vi "WSVCAP SHL Host TL RFFE Write Cycle - Single DUT.vi"(0 "Data Out (Cycle Commands)":string[](array[string]), 5 "Post Command Delay":dbl[](array[numeric]) format="%#.0p s", 11 "error in":errorcluster, 12 "Log (T)":bool=TRUE, 13 "DUT":T2, 14 "FPGA":T1) -> (15 "error out":errorcluster)   [LabVIEW 2017]
uses:
  Type Defs/WSVCAP SHL DUT Number Enum.ctl
  Type Defs/WSVCAP SHL FPGA Enum.ctl
panel:
  out "Socket Mask":u64=1 format="%016x"
  out "RFFE Data Out":u8[][](array[numeric]) format="%02x"
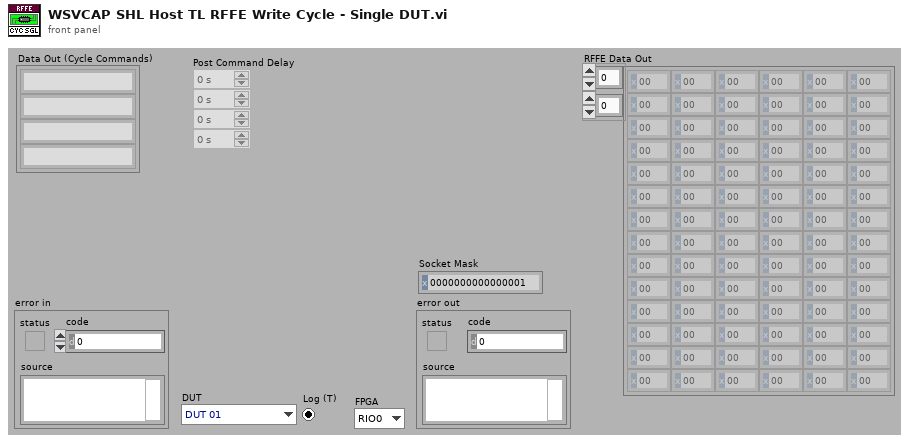
[diagram p1: front panel]
types:
  T1 = typedef "WSVCAP SHL FPGA Enum.ctl" = enum16{"RIO0", "RIO1"}
  T2 = typedef "WSVCAP SHL DUT Number Enum.ctl" = enum16{"DUT 01", "DUT 02", "DUT 03", "DUT 04", "DUT 05", "DUT 06", "DUT 07", "DUT 08", "DUT 09", "DUT 10", "DUT 11", "DUT 12", "DUT 13", "DUT 14", "DUT 15", "DUT 16", "DUT 17", "DUT 18", "DUT 19", "DUT 20", "DUT 21", "DUT 22", "DUT 23", "DUT 24", "DUT 25", "DUT 26", "DUT 27", "DUT 28", "DUT 29", "DUT 30", "DUT 31", "DUT 32", "DUT 33", "DUT 34", "DUT 35", "DUT 36", "DUT 37", "DUT 38", "DUT 39", "DUT 40", "DUT 41", "DUT 42", "DUT 43", "DUT 44", "DUT 45", "DUT 46", "DUT 47", "DUT 48", "DUT 49", "DUT 50", "DUT 51", "DUT 52", "DUT 53", "DUT 54", "DUT 55", "DUT 56", "DUT 57", "DUT 58", "DUT 59", "DUT 60", "DUT 61", "DUT 62", "DUT 63", "DUT 64"}
  T3 = typedef "WSVCAP SHL Core System Cluster.ctl" = cluster{"Settings":T4, "FPGA Resource":tag, "Online":bool, "I2C Wait Ticks":u32, "SPI Wait Ticks":u32, "RFFE Wait Ticks":u32, "FPGA VI Reference (FPGA Mode)":T5, "FPGA VI Reference (Sim Mode)":refnum<vi>}
  T4 = typedef "WSVCAP SHL I2C Settings Cluster.ctl" = cluster{"I2C Slave Address":u8, "I2C Clock Rate (Hz)":dbl, "SPI Clock Rate (Hz)":dbl, "RFFE Slave Address":u8, "RFFE Clock Rate (Hz)":dbl, "Simulate FPGA":bool, "C1 Cap DAC Default":u8, "C2 Cap DAC Default":u8, "C3 Cap DAC Default":u8, "C4 Cap DAC Default":u8}
  T5 = typedef "WSVCAP SHL FPGA Ref.ctl" = refnum<k20>
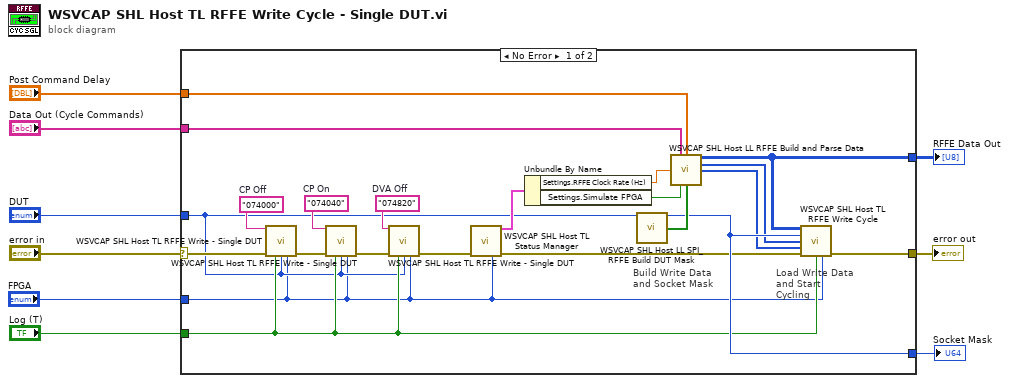
[diagram p0: block diagram]
diagram:
  n1 = case shown="No Error" "error in" {
    selector: "error in" -> [w20 _]
    tunnel: [w27 _] -> w9
    tunnel: [w11 _] -> w7
    tunnel: "DUT" -> [w12 _]
    tunnel: [w30 _] -> w5
    tunnel: "Log (T)" -> [w13 _]
    tunnel: "Post Command Delay" -> [w29 _]
    tunnel: "Data Out (Cycle Commands)" -> [w28 _]
    tunnel: "FPGA" -> [w10 _]
    frame No Error {
      w14 = "074820"  # DVA Off
      w15 = "074040"  # CP On
      w16 = "074000"  # CP Off
      # "Load Write Data and Start Cycling"
      # "Build Write Data and Socket Mask"
      n2 = call "WSVCAP SHL Host TL RFFE Write - Single DUT.vi"("Data Out"=w16, "error in"=w20, "Log (T)"=w13, "DUT"=w12, "FPGA"=w10) -> ("error out"=w19:errorcluster)  [unwired: 10 in]
      n3 = call "WSVCAP SHL Host TL RFFE Write - Single DUT.vi"("Data Out"=w15, "error in"=w19, "Log (T)"=w13, "DUT"=w12, "FPGA"=w10) -> ("error out"=w18:errorcluster)  [unwired: 10 in]
      n4 = call "WSVCAP SHL Host TL RFFE Write - Single DUT.vi"("Data Out"=w14, "error in"=w18, "Log (T)"=w13, "DUT"=w12, "FPGA"=w10) -> ("error out"=w17:errorcluster)  [unwired: 10 in]
      n5 = call "WSVCAP SHL Host TL Status Manager.vi"("error in"=w17, "FPGA"=w10) -> ("System Out"=w25:T3, "error out"=w26:errorcluster)  [unwired: 12 in]
      n6 = Unbundle By Name(w25) -> ("Settings.RFFE Clock Rate (Hz)"=w21:dbl, "Settings.Simulate FPGA"=w24:bool)
      n7 = call "WSVCAP SHL Host LL SPI_RFFE Build DUT Mask.vi"("DUT"=w12) -> ("Socket Mask [U64]"=w30:u64, "DUT Mask"=w31:bool[])  [unwired: 13 in]
      n8 = call "WSVCAP SHL Host LL RFFE Build and Parse Data.vi"("Data Out (Cycle Commands)"=w28, "Post Command Delay"=w29, "Clock Rate (Hz) (Cycle Only)"=w21, "Simulate FPGA (Cycle Only)"=w24, "DUT Mask (All)"=w31) -> ("RFFE Data Out [U8]"=w11:u8[][], "CMD Lengths (Bits)"=w23:u8[], "CMD Delays (Ticks)"=w22:u32[])  [unwired: 7 in, 1 out]
      n9 = call "WSVCAP SHL Host TL RFFE Write Cycle.vi"("RFFE Data Out"=w11, "Socket Mask"=w30, "Cycle CMD Lengths (bits)"=w23, "Cycle CMD Delay (ticks)"=w22, "error in"=w26, "Log (T)"=w13, "FPGA"=w10) -> ("error out"=w27:errorcluster)  [unwired: 8 in]
    }
    frame Error {
    }
  }
  "error out" <- w9
  "RFFE Data Out" <- w7
  "Socket Mask" <- w5
